vi "Add Channel.vi"(8 "error in":errorcluster, 10 "hardwareChannel":i32, 11 "parameter file in":refnum<k24>) -> (0 "error out":errorcluster, 2 "new channel":refnum<k24>, 3 "parameter file out":refnum<k24>)   [LabVIEW 2020, in "Ballard_429_Parameter_ni.lvlib"]
uses:
  Ballard_429_Parameter_ni.lvlib
  C:/Users/Administrator/Desktop/GIT/Ballard-Arinc-429-XML-Generator/Source/Assemblies/Ballard_429_Parameter_ni/bin/Debug/Ballard_429_Parameter_ni.dll
  Assemblies/Ballard_429_Parameter_ni/bin/Debug/Ballard_429_Parameter_ni.dll
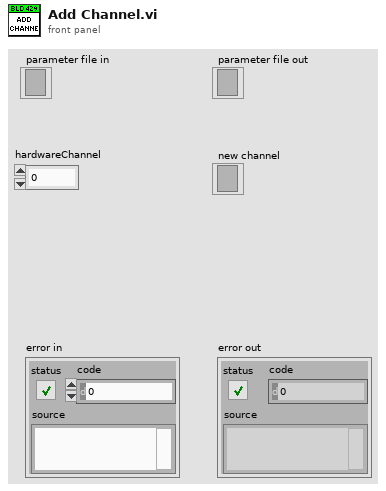
[diagram p1: front panel]
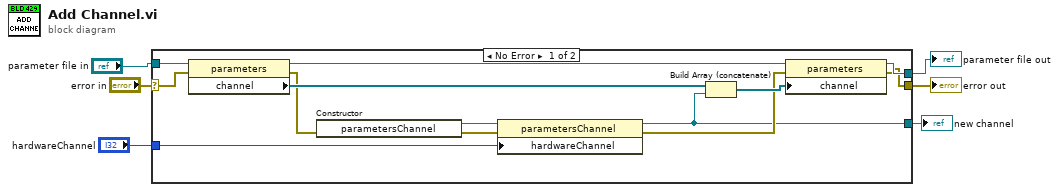
[diagram p0: block diagram]
diagram:
  n1 = case shown="No Error" "error in" {
    selector: "error in" -> [w18 w20]
    tunnel: [w14 w21] -> w6
    tunnel: [w13 w20] -> w5
    tunnel: "parameter file in" -> [w19 w21]
    tunnel: [w8 _] -> w2
    tunnel: "hardwareChannel" -> [w7 _]
    frame No Error {
      n2 = property class="parameters"(reference=w19, error in=w18) -> (reference out=w15:refnum<k24>, error out=w16:errorcluster, "channel"=w17:refnum<k24>[])
      n3 = constructor class="parametersChannel"(error in=w16) -> (reference out=w11:refnum<k24>, error out=w10:errorcluster)  [unwired: 2 in, 1 out]
      n4 = property class="parametersChannel"(reference=w11, error in=w10, "hardwareChannel"=w7) -> (reference out=w8:refnum<k24>, error out=w9:errorcluster)
      n5 = Build Array (concatenate)(w17, w8) -> (w12:refnum<k24>[])
      n6 = property class="parameters"(reference=w15, error in=w9, "channel"=w12) -> (reference out=w14:refnum<k24>, error out=w13:errorcluster)
    }
    frame Error {
    }
  }
  "parameter file out" <- w6
  "error out" <- w5
  "new channel" <- w2
